vi "ThermalProfile_interface.vi"() -> ()   [LabVIEW 2016]
uses:
  <vilib>/httpClient/ClientHandle.ctl
  Type_Defs/Digital_Out.ctl
  Type_Defs/Digital_In_1.ctl
  Type_Defs/Analog_In.ctl
  msg7171_linux.llb/send single message.vi
  <vilib>/httpClient/POSTBuffer.vi
  <vilib>/httpClient/LabVIEWHTTPClient.lvlib
  msg7171_linux.llb/send multiple messages.vi
panel:
  in  "Cluster 2":cluster{"Step #":u32, "Soak Temp":dbl} {"Soak Temp" min=0.0 max=10080.0 step=0.1}
  in  "Cluster":T1 {"Soak Duration" min=0.0 max=10080.0 step=0.1; "Ramp Duration" min=0.0 max=10080.0 step=0.1}
  in  "Scrollbar":i32(c297)
  in  "exit":bool
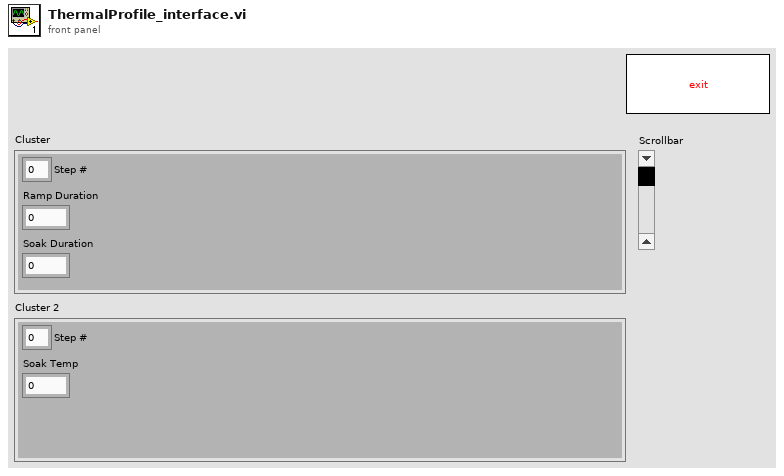
[diagram p1: front panel]
types:
  T1 = cluster{"Step #":u32, "Ramp Duration":dbl, "Soak Duration":dbl}
  T2 = typedef "LabVIEWHTTPClient.lvlib/ClientHandle.ctl" = refnum<k1>
  T3 = cluster{"go":bool, "Http session":T2, "URL prefex":string}
  T4 = typedef "Digital_Out.ctl" = cluster{"LN2-P EN":bool, "LN2-S EN":bool, "LN2-Sol EN":bool, "IR Lamp 1":bool, "IR Lamp 2":bool, "IR Lamp 3":bool, "IR Lamp 4":bool, "IR Lamp 5":bool, "IR Lamp 6":bool, "IR Lamp 7":bool, "IR Lamp 8":bool, "IR Lamp 9":bool, "IR Lamp 10":bool, "IR Lamp 11":bool, "IR Lamp 12":bool, "IR Lamp 13":bool, "IR Lamp 14":bool, "IR Lamp 15":bool, "IR Lamp 16":bool, "Heater SSR 1":bool, "Heater SSR 2":bool, "Heater SSR 3":bool, "Heater SSR 4":bool, "Heater SSR 5":bool, "Heater SSR 6":bool, "Heater SSR 7":bool, "Heater SSR 8":bool, "Heater SSR 9":bool, "Heater SSR 10":bool, "Heater SSR 11":bool, "Heater SSR 12":bool, "Heater SSR 13":bool, "Heater SSR 14":bool, "Heater SSR 15":bool, "Heater SSR 16":bool, "Heater SSR 17":bool, "Heater SSR 18":bool, "Heater SSR 19":bool, "Heater SSR 20":bool, "Heater SSR 21":bool, "MCC Power":bool, "MCC2 Power":bool, "RoughP GateValve":bool, "RoughP Start":bool, "CryoP GateValve":bool, "RoughP PurgeGass":bool, "LN2-S Sol":bool, "LN2-P Sol":bool, "CryoP Pwr Relay 1":bool, "CryoP Pwr Relay 2":bool, "RoughP Pwr Relay":bool}
  T5 = typedef "Digital_In_1.ctl" = cluster{"PG-SW-RoughP-Relay 1":bool, "PG-SW-RoughP-Relay 2":bool, "PG-SW-CryoP-Relay 1":bool, "PG-SW-CryoP-Relay 2":bool, "PG-SW-Chamber-Relay 1":bool, "PG-SW-Chamber-Relay 2":bool, "LN2-P-Sol-Open: NC":bool, "LN2-P-Sol-Open: O":bool, "LN2-P-Sol-Closed: NC":bool, "LN2-P-Sol-Closed: O":bool, "LN2-S-Sol-Open: NC":bool, "LN2-S-Sol-Open: O":bool, "LN2-S-Sol-Closed: NC":bool, "LN2-S-Sol-Closed: O":bool, "CryoP-GV-Open: NC":bool, "CryoP-GV-Open: O":bool, "CryoP-GV-Closed: NC":bool, "CryoP-GV-Closed: O":bool, "RoughP-GV-Open":bool, "RoughP-GV-Closed":bool, "RoughP-Pwr: NC":bool, "RoughP-Pwr: O":bool, "RoughP-On: NC":bool, "RoughP-On: O":bool, "Air supply LN2 OK":bool, "Air supply OK":bool}
  T6 = typedef "Analog_In.ctl" = cluster{"Cabinet Temp 1":u16, "Cabinet Temp 2":u16, "Cabinet Temp 3":u16, "fs Front Door 1":u16, "fs Front Door 2":u16, "fs Front Door 3":u16, "fs Back Door 1":u16, "fs Back Door 2":u16, "fs Back Door 3":u16, "Rough Pump Temp":u16, "pg Chamber":u16, "pg Cryo Pump":u16, "pg Rough Pump":u16, "LN2 platen":u16, "LN2 shroud":u16}
  T7 = cluster{"out":cluster{"LN2 Platen":u16, "LN2 Shroud":u16}, "in":T6}
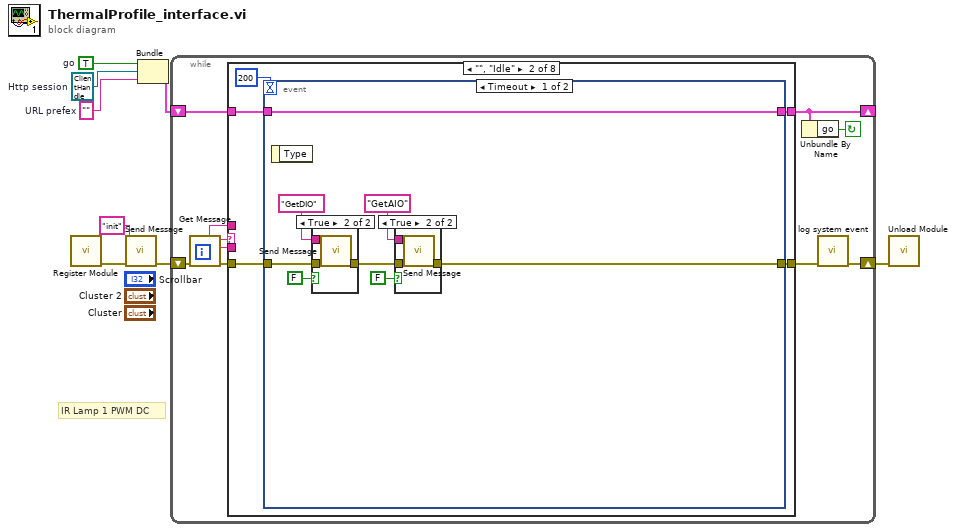
[diagram p0: block diagram]
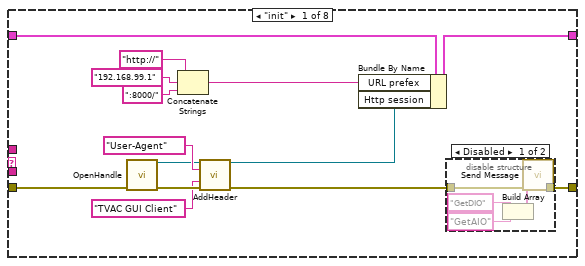
[diagram p2: hidden frame]
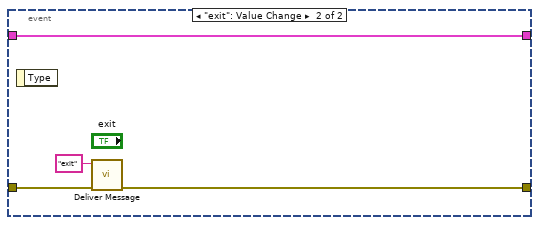
[diagram p6: hidden frame]
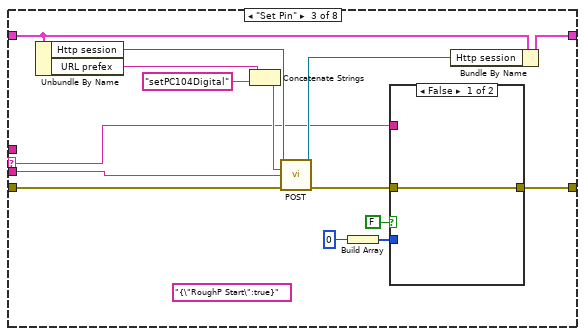
[diagram p7: hidden frame]
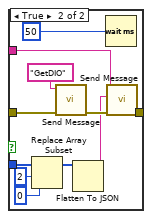
[diagram p8: hidden frame]
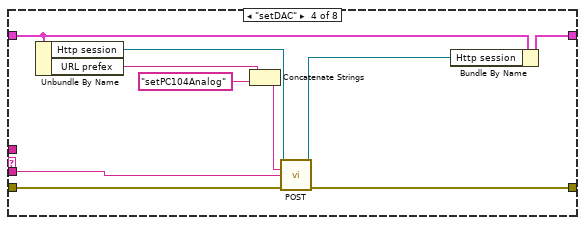
[diagram p9: hidden frame]
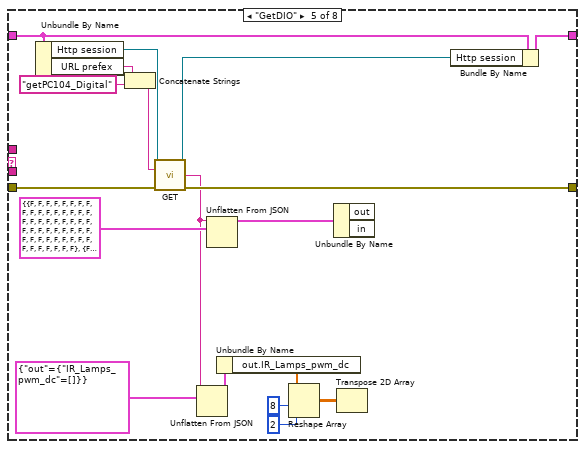
[diagram p10: hidden frame]
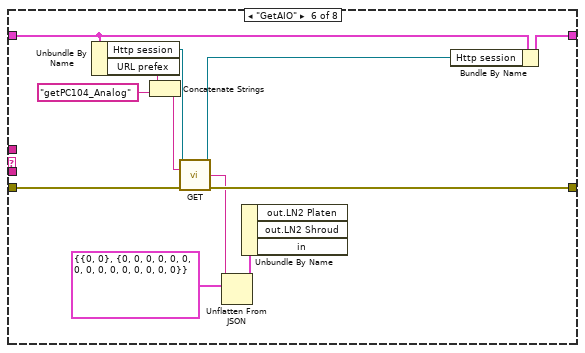
[diagram p11: hidden frame]
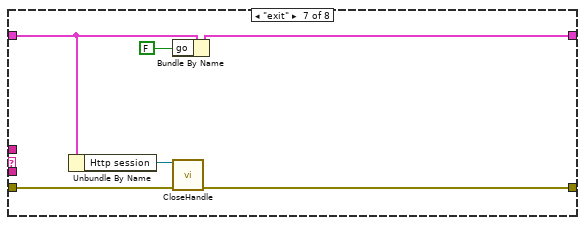
[diagram p12: hidden frame]
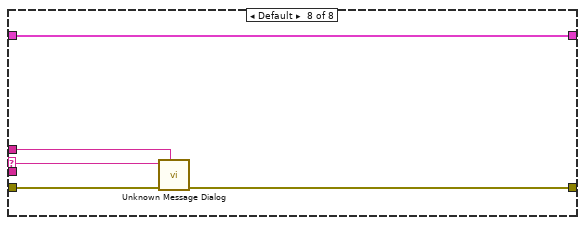
[diagram p13: hidden frame]
diagram:
  w4 = ""  # URL prefex
  w5 = T2 refnum  # Http session
  w6 = TRUE  # go
  # "IR Lamp 1 PWM DC"
  n1 = call "Register Module.vi"() -> ("error out"=w2:errorcluster)  [unwired: 10 in, 1 out]
  n2 = call-poly "Send Message.vi"("error in (no error)"=w2, "event"="init") -> ("error out"=w1:errorcluster)  [unwired: 9 in]
  n3 = Bundle("go"=w6, "Http session"=w5, "URL prefex"=w4) -> (w8:T3)  [unwired: 1 in]
  n4 = while {
    shift-left: w8 -> [w15]
    shift-right: [w12] -> _
    shift-right: [w10] -> w7
    shift-left: w1 -> [w18]
    stop <- w11 continue-if-true
    n5 = call "Get Message.vi"("error in (no error)"=w18) -> ("error out"=w16:errorcluster, "event buffer"=w17:string, "event"=w14:string, "source"=w13:string)  [unwired: 7 in]
    n6 = case shown="\"\", \"Idle\"" w14 {
      selector: w14 -> [_ _ w69 _ _ _ _ w139]
      tunnel: [w23 w40 w73 w95 w111 w123 w136 w141] -> w12
      tunnel: w15 -> [w32 w39 w72 w94 w110 w122 w131 w141]
      tunnel: w17 -> [_ _ w67 w91 _ _ _ _]
      tunnel: w16 -> [w27 w41 w71 w93 w113 w125 w134 w140]
      tunnel: w13 -> [_ _ _ _ _ _ _ w138]
      tunnel: [w19 w43 w70 w92 w112 w124 w133 w137] -> w9
      frame "init" {
        n7 = call <vilib>:"OpenHandle.vi"("error in (no error)"=w27) -> ("client handle out"=w28:T2, "error out"=w31:errorcluster)  [unwired: 13 in]
        n8 = Concatenate Strings("http://" ("url"), "192.168.99.1" ("Address"), ":8000/" ("url")) -> (w22:string)
        n9 = call <vilib>:"AddHeader.vi"("client handle"=w28, "header"="User-Agent", "value"="TVAC GUI Client", "error in (no error)"=w31) -> ("client handle out"=w21:T2, "error out"=w20:errorcluster)  [unwired: 10 in]
        n10 = Bundle By Name(cluster=w32, "URL prefex"=w22, "Http session"=w21) -> (w23:T3)
        n11 = disable-structure shown="Disabled" {
          disable-tunnel: w20 -> [w37 w38]
          disable-tunnel: [w36 w38] -> w19
          frame Disabled {
            n12 = Build Array("GetDIO" ("event"), "GetAIO" ("event")) -> (w34:string[])
            n13 = call-poly "Send Message.vi"("error in (no error)"=w37, "event"=w34) -> ("error out"=w36:errorcluster)  [unwired: 9 in]
          }
          frame Enabled {
          }
        }
      }
      frame "", "Idle" {
        n14 = event shown="[0] Timeout" {
          selector: _ -> [_ _]
          dyn-events: _ -> [_ _]
          timeout: 200 ("milliseconds to wait") -> [_ _]
          tunnel: w41 -> [w50 w63]
          tunnel: [w46 w62] -> w43
          tunnel: [w51 w60] -> w40
          tunnel: w39 -> [w51 w60]
          event Timeout {
            n15 = event-data() -> ()  [unwired: 1 in, 1 out]
            n16 = case shown="True" FALSE {
              tunnel: w50 -> [w56 w59]
              tunnel: [w56 w58] -> w48
              tunnel: "GetDIO" ("event") -> [_ w57]
              frame False {
              }
              frame True {
                n17 = call-poly "Send Message.vi"("error in (no error)"=w59, "event"=w57) -> ("error out"=w58:errorcluster)  [unwired: 9 in]
              }
            }
            n18 = case shown="True" FALSE {
              tunnel: w48 -> [w52 w55]
              tunnel: [w52 w54] -> w46
              tunnel: "GetAIO" ("event") -> [_ w53]
              frame False {
              }
              frame True {
                n19 = call-poly "Send Message.vi"("error in (no error)"=w55, "event"=w53) -> ("error out"=w54:errorcluster)  [unwired: 9 in]
              }
            }
          }
          event "exit": Value Change {
            n20 = event-data() -> ()  [unwired: 1 in, 1 out]
            n21 = call "Deliver Message.vi"("error in (no error)"=w63, "event"="exit") -> ("error out"=w62:errorcluster)  [unwired: 9 in]
          }
        }
      }
      frame "Set Pin" {
        (unwired) "{\"RoughP Start\":true}" ("string")
        n22 = Unbundle By Name(w72) -> ("Http session"=w77:T2, "URL prefex"=w75:string)
        n23 = Concatenate Strings(w75, "setPC104Digital" ("url")) -> (w76:string)
        n24 = call-poly <vilib>:"POST.vi"("client handle"=w77, "url"=w76, "buffer"=w67, "error in (no error)"=w71) -> ("client handle out"=w78:T2, "error out"=w68:errorcluster)  [unwired: 8 in, 2 out]
        n25 = Build Array(0) -> (w65:i32[])
        n26 = case shown="False" FALSE {
          tunnel: [w79 w90] -> w70
          tunnel: w69 -> [_ w89]
          tunnel: w68 -> [w79 w88]
          tunnel: w65 -> [_ w85]
          frame False {
          }
          frame True {
            n27 = Replace Array Subset(array=w85, new element=0 ("new element/subarray"), index=2) -> (w81:i32[])
            n28 = call-poly "Send Message.vi"("error in (no error)"=w88, "event"="GetDIO") -> ("error out"=w87:errorcluster)  [unwired: 9 in]
            n29 = Flatten To JSON(anything=w81) -> (JSON string=w82:string)  [unwired: 2 in, 1 out]
            n30 = Wait (ms)(milliseconds to wait=u32 50) -> ()  [unwired: 1 out]
            n31 = call-poly "Send Message.vi"("error in (no error)"=w87, "event buffer"=w82, "event"=w89) -> ("error out"=w90:errorcluster)  [unwired: 8 in]
          }
        }
        n32 = Bundle By Name(cluster=w72, "Http session"=w78) -> (w73:T3)
      }
      frame "setDAC" {
        n33 = Unbundle By Name(w94) -> ("Http session"=w99:T2, "URL prefex"=w97:string)
        n34 = Concatenate Strings(w97, "setPC104Analog" ("url")) -> (w98:string)
        n35 = call-poly <vilib>:"POST.vi"("client handle"=w99, "url"=w98, "buffer"=w91, "error in (no error)"=w93) -> ("client handle out"=w100:T2, "error out"=w92:errorcluster)  [unwired: 8 in, 2 out]
        n36 = Bundle By Name(cluster=w94, "Http session"=w100) -> (w95:T3)
      }
      frame "GetDIO" {
        n37 = Unbundle By Name(w110) -> ("Http session"=w117:T2, "URL prefex"=w115:string)
        n38 = Concatenate Strings(w115, "getPC104_Digital" ("url")) -> (w116:string)
        n39 = call <vilib>:"GET.vi"("client handle"=w117, "url"=w116, "error in (no error)"=w113) -> ("client handle out"=w118:T2, "body"=w101:string, "error out"=w112:errorcluster)  [unwired: 9 in, 1 out]
        n40 = Unflatten From JSON(JSON string=w101, type and defaults=cluster{"out":cluster{"IR_Lamps_pwm_dc":dbl[]}} {"out"={"IR_Lamps_pwm_dc"=[]}}) -> (value=w103:cluster{"out":cluster{"IR_Lamps_pwm_dc":dbl[]}})  [unwired: 5 in, 1 out]
        n41 = Unflatten From JSON(JSON string=w101, type and defaults=cluster{"out":T4, "in":T5} {"out"={"LN2-P EN"=FALSE, "LN2-S EN"=FALSE, "LN2-Sol EN"=FALSE, "IR Lamp 1"=FALSE, "IR Lamp 2"=FALSE, "IR Lamp 3"=FALSE, "IR Lamp 4"=FALSE, "IR Lamp 5"=FALSE, "IR Lamp 6"=FALSE, "IR Lamp 7"=FALSE, "IR Lamp 8"=FALSE, "IR Lamp 9"=FALSE, "IR Lamp 10"=FALSE, "IR Lamp 11"=FALSE, "IR Lamp 12"=FALSE, "IR Lamp 13"=FALSE, "IR Lamp 14"=FALSE, "IR Lamp 15"=FALSE, "IR Lamp 16"=FALSE, "Heater SSR 1"=FALSE, "Heater SSR 2"=FALSE, "Heater SSR 3"=FALSE, "Heater SSR 4"=FALSE, "Heater SSR 5"=FALSE, "Heater SSR 6"=FALSE, "Heater SSR 7"=FALSE, "Heater SSR 8"=FALSE, "Heater SSR 9"=FALSE, "Heater SSR 10"=FALSE, "Heater SSR 11"=FALSE, "Heater SSR 12"=FALSE, "Heater SSR 13"=FALSE, "Heater SSR 14"=FALSE, "Heater SSR 15"=FALSE, "Heater SSR 16"=FALSE, "Heater SSR 17"=FALSE, "Heater SSR 18"=FALSE, "Heater SSR 19"=FALSE, "Heater SSR 20"=FALSE, "Heater SSR 21"=FALSE, "MCC Power"=FALSE, "MCC2 Power"=FALSE, "RoughP GateValve"=FALSE, "RoughP Start"=FALSE, "CryoP GateValve"=FALSE, "RoughP PurgeGass"=FALSE, "LN2-S Sol"=FALSE, "LN2-P Sol"=FALSE, "CryoP Pwr Relay 1"=FALSE, "CryoP Pwr Relay 2"=FALSE, "RoughP Pwr Relay"=FALSE}, "in"={"PG-SW-RoughP-Relay 1"=FALSE, "PG-SW-RoughP-Relay 2"=FALSE, "PG-SW-CryoP-Relay 1"=FALSE, "PG-SW-CryoP-Relay 2"=FALSE, "PG-SW-Chamber-Relay 1"=FALSE, "PG-SW-Chamber-Relay 2"=FALSE, "LN2-P-Sol-Open: NC"=FALSE, "LN2-P-Sol-Open: O"=FALSE, "LN2-P-Sol-Closed: NC"=FALSE, "LN2-P-Sol-Closed: O"=FALSE, "LN2-S-Sol-Open: NC"=FALSE, "LN2-S-Sol-Open: O"=FALSE, "LN2-S-Sol-Closed: NC"=FALSE, "LN2-S-Sol-Closed: O"=FALSE, "CryoP-GV-Open: NC"=FALSE, "CryoP-GV-Open: O"=FALSE, "CryoP-GV-Closed: NC"=FALSE, "CryoP-GV-Closed: O"=FALSE, "RoughP-GV-Open"=FALSE, "RoughP-GV-Closed"=FALSE, "RoughP-Pwr: NC"=FALSE, "RoughP-Pwr: O"=FALSE, "RoughP-On: NC"=FALSE, "RoughP-On: O"=FALSE, "Air supply LN2 OK"=FALSE, "Air supply OK"=FALSE}}) -> (value=w108:cluster{"out":T4, "in":T5})  [unwired: 5 in, 1 out]
        n42 = Unbundle By Name(w103) -> ("out.IR_Lamps_pwm_dc"=w102:dbl[])
        n43 = Reshape Array(w102, 8 ("dimension size"), 2 ("dimension size")) -> (w105:dbl[][])
        n44 = Unbundle By Name(w108) -> ()  [unwired: 2 out]
        n45 = Transpose 2D Array(2D array=w105) -> ()  [unwired: 1 out]
        n46 = Bundle By Name(cluster=w110, "Http session"=w118) -> (w111:T3)
      }
      frame "GetAIO" {
        n47 = Unbundle By Name(w122) -> ("Http session"=w129:T2, "URL prefex"=w127:string)
        n48 = Concatenate Strings(w127, "getPC104_Analog" ("url")) -> (w128:string)
        n49 = call <vilib>:"GET.vi"("client handle"=w129, "url"=w128, "error in (no error)"=w125) -> ("client handle out"=w130:T2, "body"=w119:string, "error out"=w124:errorcluster)  [unwired: 9 in, 1 out]
        n50 = Unflatten From JSON(JSON string=w119, type and defaults=T7 {"out"={"LN2 Platen"=0, "LN2 Shroud"=0}, "in"={"Cabinet Temp 1"=0, "Cabinet Temp 2"=0, "Cabinet Temp 3"=0, "fs Front Door 1"=0, "fs Front Door 2"=0, "fs Front Door 3"=0, "fs Back Door 1"=0, "fs Back Door 2"=0, "fs Back Door 3"=0, "Rough Pump Temp"=0, "pg Chamber"=0, "pg Cryo Pump"=0, "pg Rough Pump"=0, "LN2 platen"=0, "LN2 shroud"=0}}) -> (value=w120:T7)  [unwired: 5 in, 1 out]
        n51 = Unbundle By Name(w120) -> ()  [unwired: 3 out]
        n52 = Bundle By Name(cluster=w122, "Http session"=w130) -> (w123:T3)
      }
      frame "exit" {
        n53 = Unbundle By Name(w131) -> ("Http session"=w132:T2)
        n54 = Bundle By Name(cluster=w131, "go"=FALSE ("Bundle Element")) -> (w136:T3)
        n55 = call <vilib>:"CloseHandle.vi"("client handle"=w132, "error in (no error)"=w134) -> ("error out"=w133:errorcluster)  [unwired: 13 in]
      }
      frame Default {
        n56 = call "Unknown Message Dialog.vi"("source"=w138, "error in (no error)"=w140, "event name"=w139) -> ("error out"=w137:errorcluster)  [unwired: 8 in]
      }
    }
    n57 = Unbundle By Name(w12) -> ("go"=w11:bool)
    n58 = call "log system event.vi"("error in (no error)"=w9) -> ("error out"=w10:errorcluster)  [unwired: 9 in, 1 out]
  }
  n59 = call "Unload Module.vi"("error in (no error)"=w7) -> ()  [unwired: 10 in, 1 out]
